vi "GUILib.simple boolean update.vi"(0 "ctlRef":refnum<vi>, 1 "isNominal":bool, 2 "value":bool, 4 "valueStatus":T1, 5 "error in (no error)":errorcluster) -> (14 "ctlRef dup":refnum<vi>, 19 "error out":errorcluster)   [LabVIEW 2012, in "GUILib.lvlib"]
doc: "updates a value for a specific type of control"
uses:
  GUILib.lvlib
  UtilityLib/UtilityLib.valueStatus.ctl
  UtilityLib/UtilityLib.lvlib
panel:
  in  "booleanType":bool
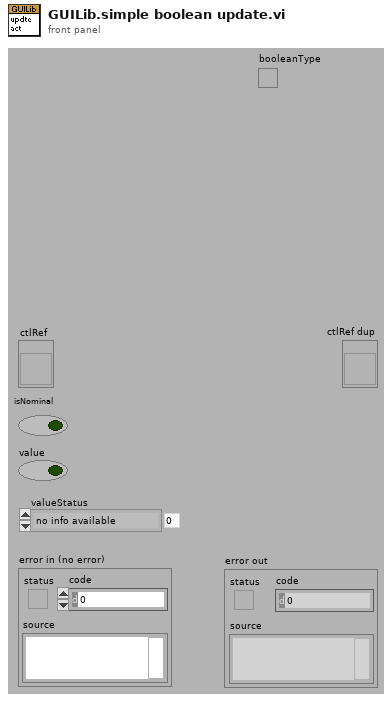
[diagram p1: front panel]
types:
  T1 = typedef "UtilityLib.lvlib/UtilityLib.valueStatus.ctl" = enum16{"no info available", "stand by/off", "on", "warning", "alarm/malfunction", "not implemented", "user action required", "important information", "system default", "control default", "indicator default", "button default"}
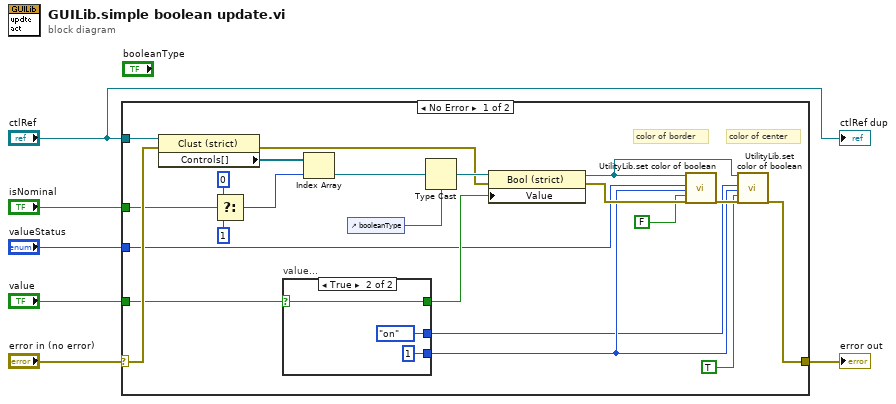
[diagram p0: block diagram]
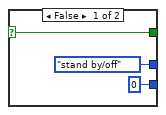
[diagram p2: hidden frame]
diagram:
  n1 = case shown="No Error" "error in (no error)" {
    selector: "error in (no error)" -> [w23 w35]
    tunnel: "ctlRef" -> [w25 _]
    tunnel: "valueStatus" -> [w12 _]
    tunnel: "value" -> [w16 _]
    tunnel: [w9 w35] -> w3
    tunnel: "isNominal" -> [w20 _]
    frame No Error {
      # "color of center"
      # "color of border"
      n2 = property on="Property Node" class="Clust (strict)"(reference=w25, error in=w23) -> (error out=w22:errorcluster, "Controls[]"=w26:refnum<vi>[])  [unwired: 1 out]
      n3 = Select(t=0, s=w20, f=1 ("index")) -> (s? t:f=w17:i32)
      n4 = case "value..." shown="True" w16 {
        selector: w16 -> [w31 w34]
        tunnel: [0 ("nOfPair (0)") 1 ("nOfPair (0)")] -> w11
        tunnel: [w31 w34] -> w15
        tunnel: [UtilityLib.valueStatus."stand by/off" ("valueStatus") UtilityLib.valueStatus."on" ("valueStatus")] -> w8
        frame False {
        }
        frame True {
        }
      }
      n5 = Index Array(array=w26, index=w17) -> (element=w27:refnum<vi>)
      n6 = control-ref of="booleanType"() -> (w28:refnum<vi>)
      n7 = Type Cast(type=w28, x=w27) -> (*(type *) &x=w24:refnum<vi>)
      n8 = property on="Property Node" class="Bool (strict)"(reference=w24, error in=w22, "Value"=w15) -> (reference out=w13:refnum<vi>, error out=w21:errorcluster)
      n9 = call "UtilityLib.set color of boolean.vi"("button"=w13, "valueStatus"=w12, "nOfPair (0)"=w11, "setTRUEColor (FALSE)"=FALSE, "error in (no error)"=w21) -> ("error out"=w14:errorcluster)  [unwired: 14 in]
      n10 = call "UtilityLib.set color of boolean.vi"("button"=w13, "valueStatus"=w8, "nOfPair (0)"=w11, "setTRUEColor (FALSE)"=TRUE, "error in (no error)"=w14) -> ("error out"=w9:errorcluster)  [unwired: 14 in]
    }
    frame Error {
    }
  }
  "error out" <- w3
  "ctlRef dup" <- "ctlRef"
